vi "Shift coordinates (SLM to IMAQ).vi"(4 "I":sgl[](array[numeric]), 5 "trap cluster in in":T1, 6 "Z":sgl[](array[numeric]), 7 "X":sgl[](array[numeric]), 9 "Y":sgl[](array[numeric]), 10 "Coordinate mapping \n(IMAQ to SLM)":T2, 11 "Number of Rows":u32) -> (3 "trap cluster in out":T1)   [LabVIEW 2011]
uses:
  Trap cluster.ctl
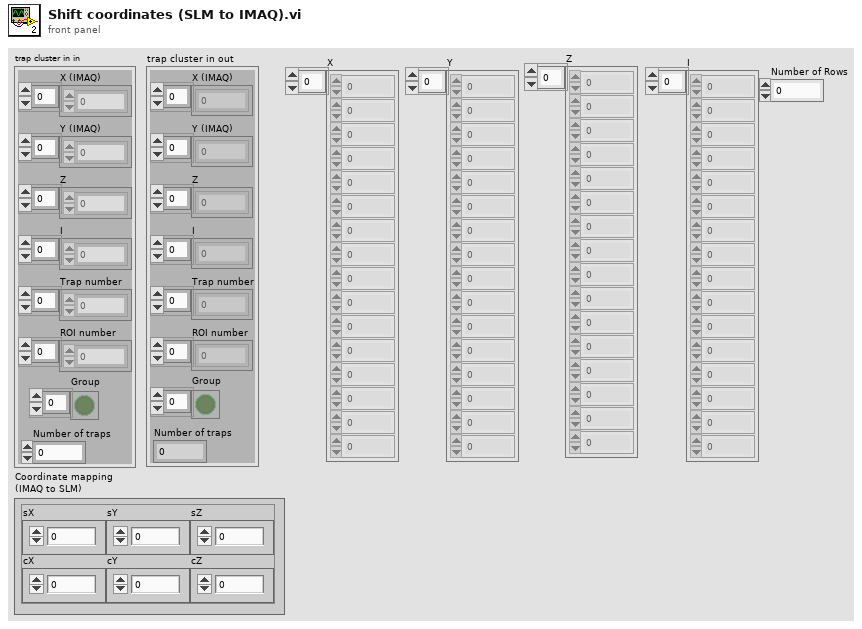
[diagram p1: front panel]
types:
  T1 = typedef "Trap cluster.ctl" = cluster{"X (IMAQ)":sgl[], "Y (IMAQ)":sgl[], "Z":sgl[], "I":sgl[], "Trap number":i32[], "ROI number":i32[], "Number of traps":i32, "Group":bool[]}
  T2 = cluster{"cZ":sgl, "cY":sgl, "cX":sgl, "sZ":sgl, "sY":sgl, "sX":sgl}
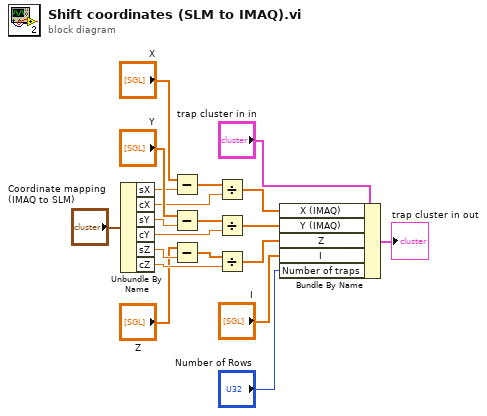
[diagram p0: block diagram]
diagram:
  n1 = Unbundle By Name("Coordinate mapping \n(IMAQ to SLM)") -> ("sX"=w8:sgl, "cX"=w9:sgl, "sY"=w11:sgl, "cY"=w14:sgl, "sZ"=w16:sgl, "cZ"=w19:sgl)
  n2 = Subtract(x="X", y=w8) -> (x-y=w5:sgl[])
  n3 = Subtract(x="Y", y=w11) -> (x-y=w13:sgl[])
  n4 = Subtract(x="Z", y=w16) -> (x-y=w18:sgl[])
  n5 = Divide(x=w5, y=w9) -> (x/y=w6:sgl[])
  n6 = Divide(x=w13, y=w14) -> (x/y=w12:sgl[])
  n7 = Divide(x=w18, y=w19) -> (x/y=w17:sgl[])
  n8 = Bundle By Name(cluster="trap cluster in in", "X (IMAQ)"=w6, "Y (IMAQ)"=w12, "Z"=w17, "I"="I", "Number of traps"="Number of Rows") -> (→"trap cluster in out":T1)
